vi "GetPrivateQueueMessage.vi"(8 "error in (no error)":errorcluster, 11 "Generator":refnum<class "Generator.lvclass">) -> (0 "error out":errorcluster, 3 "Generator out":refnum<class "Generator.lvclass">)   [LabVIEW 2019, in "Generator.lvclass"]
uses:
  Generator.lvclass
  typedefs/Message--Cluster.ctl
panel:
  out "Message":T1
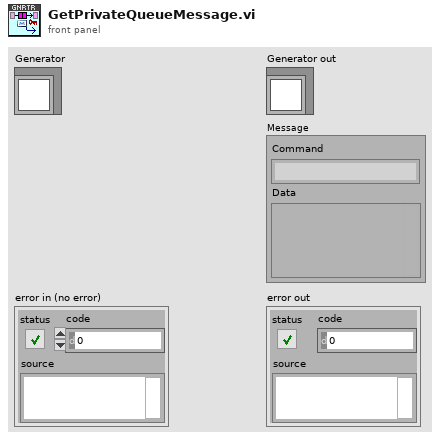
[diagram p1: front panel]
types:
  T1 = typedef "Generator.lvclass/Message--Cluster.ctl" = cluster{"Command":string, "Data":variant}
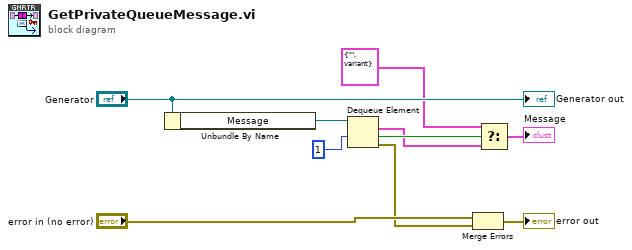
[diagram p0: block diagram]
diagram:
  n1 = Unbundle By Name("Generator") -> ("Message"=w10:refnum<queue>)
  n2 = Dequeue Element(queue=w10, timeout in ms (-1)=1) -> (element=w5:T1, timed out?=w9:bool, error out=w7:errorcluster)  [unwired: 1 in, 1 out]
  n3 = Merge Errors("error in (no error)", w7) -> (→"error out":errorcluster)
  n4 = Select(t=T1 {"Command"="", "Data"=variant}, s=w9, f=w5) -> (s? t:f=→"Message":T1)
  "Generator out" <- "Generator"
